vi "Read Command.vi"(6 "abort (F)":bool, 7 "timeout in ms (-1)":i32=-1, 8 "GUID":string, 9 "ack id (0)":u32, 10 "channel":T1) -> (0 "last element?":bool, 1 "remaining":i32, 2 "element":T2, 3 "element valid?":bool, 4 "aborted?":bool, 5 "timed out?":bool)   [LabVIEW 2019, in "MessengerM.lvlib"]
doc: "Reads a command from a Messenger channel or signals the channel to abort. This endpoint is the same as the Read endpoint except that it has an <B>abort</B> input and an <B>aborted?</B> output. You can use the abort capability of the Messenger channel to close a channel abruptly, ignoring any data left in the channel buffer. You must use this endpoint together with the Write With Abort endpoint."
uses:
  MessengerM.lvlib
  Element.ctl
  ))Channel.ctl
  ParmsIn.ctl
  EndpointOp.ctl
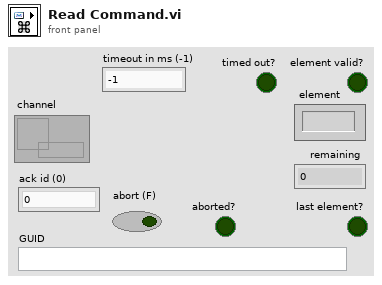
[diagram p1: front panel]
types:
  T1 = typedef "MessengerM.lvlib/))Channel.ctl" = refnum<queue>
  T2 = typedef "MessengerM.lvlib/Element.ctl" = string
  T3 = typedef "MessengerM.lvlib/ParmsIn.ctl" = cluster{"subchannel":i32, "size (0)":i32, "abort (F)":bool, "timeout":i32, "ack id (0)":u32, "last elt? (F)":bool, "valid? (T)":bool, "GUID":string}
  T4 = typedef "MessengerM.lvlib/EndpointOp.ctl" = enum16{"Write", "WriteAck", "WriteSync", "Read", "ReadAck"}
  T5 = typedef "MessengerM.lvlib/ParmsOut.ctl" = cluster{"count":i32, "aborted?":bool, "timedout?":bool, "id":u32, "last elt?":bool, "valid?":bool}
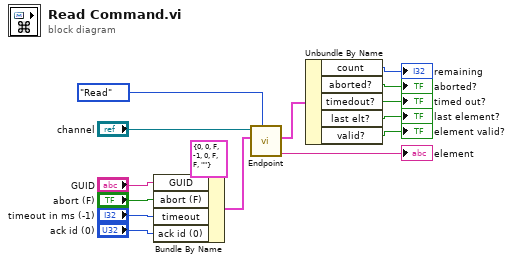
[diagram p0: block diagram]
diagram:
  n1 = Bundle By Name(cluster=T3 {"subchannel"=0, "size (0)"=0, "abort (F)"=FALSE, "timeout"=-1, "ack id (0)"=0, "last elt? (F)"=FALSE, "valid? (T)"=FALSE, "GUID"=""} ("parms in"), "GUID"="GUID", "abort (F)"="abort (F)", "timeout"="timeout in ms (-1)", "ack id (0)"="ack id (0)") -> (w8:T3)
  n2 = call "Endpoint.vi"("endpointOp"=EndpointOp."Read", "parms in"=w8, "channel in"="channel") -> ("element out"=→"element":T2, "parms out"=w3:T5)  [unwired: 7 in]
  n3 = Unbundle By Name(w3) -> ("count"=→"remaining":i32, "aborted?"=→"aborted?":bool, "timedout?"=→"timed out?":bool, "last elt?"=→"last element?":bool, "valid?"=→"element valid?":bool)
